vi "status.vi"(6 "tab sheet":T1(ring), 7 "TDMS File Viewer Configuration":T2) -> (3 "status":string)   [LabVIEW 2020]
uses:
  <vilib>/Utility/tdmsutil.llb/fileViewerConfigData.ctl
  <vilib>/Utility/tdmsutil.llb/TDMSFileViewerLocalizedText.vi
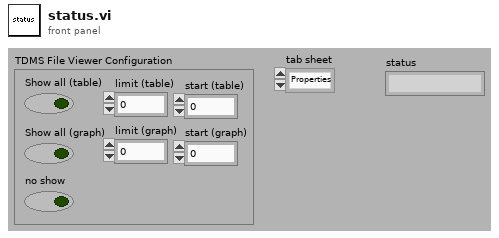
[diagram p1: front panel]
types:
  T1 = enum32{"Properties", "Values (table)", "Analog values (graph)"}
  T2 = typedef "fileViewerConfigData.ctl" = cluster{"Show all (table)":bool, "Show all (graph)":bool, "limit (table)":u64, "limit (graph)":u64, "no show":bool, "start (table)":u64, "start (graph)":u64}
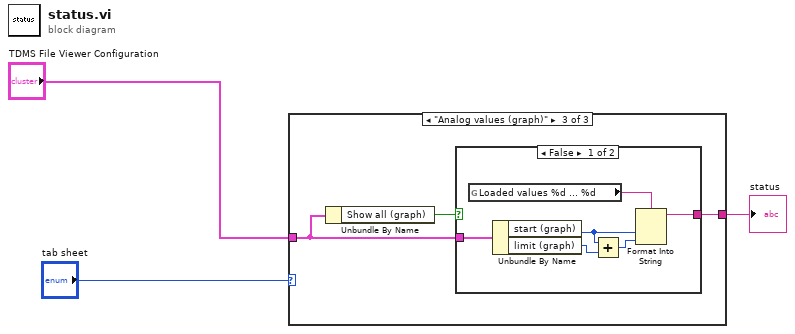
[diagram p0: block diagram]
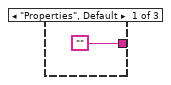
[diagram p2: hidden frame]
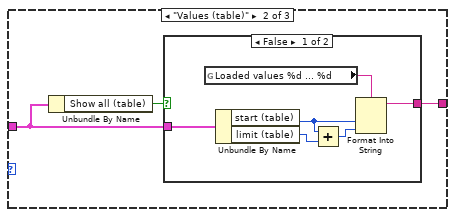
[diagram p3: hidden frame]
diagram:
  n1 = case shown="\"Analog values (graph)\"" "tab sheet" {
    tunnel: ["" w7 w16] -> w2
    tunnel: "TDMS File Viewer Configuration" -> [_ w6 w15]
    frame "Properties", Default {
    }
    frame "Values (table)" {
      n2 = Unbundle By Name(w6) -> ("Show all (table)"=w5:bool)
      n3 = case shown="False" w5 {
        tunnel: w6 -> [w13 _]
        tunnel: [w9 _] -> w7
        frame False {
          n4 = global read "TDMSFileViewerLocalizedText.vi" "Loaded values %d ... %d"() -> (w8:string)
          n5 = Unbundle By Name(w13) -> ("start (table)"=w12:u64, "limit (table)"=w11:u64)
          n6 = Add(x=w12, y=w11) -> (x+y=w10:u64)
          n7 = Format Into String(format string=w8, w12, w10) -> (resulting string=w9:string)  [unwired: 2 in, 1 out]
        }
        frame True {
        }
      }
    }
    frame "Analog values (graph)" {
      n8 = Unbundle By Name(w15) -> ("Show all (graph)"=w14:bool)
      n9 = case shown="False" w14 {
        tunnel: w15 -> [w22 _]
        tunnel: [w18 _] -> w16
        frame False {
          n10 = global read "TDMSFileViewerLocalizedText.vi" "Loaded values %d ... %d"() -> (w17:string)
          n11 = Unbundle By Name(w22) -> ("start (graph)"=w21:u64, "limit (graph)"=w20:u64)
          n12 = Add(x=w21, y=w20) -> (x+y=w19:u64)
          n13 = Format Into String(format string=w17, w21, w19) -> (resulting string=w18:string)  [unwired: 2 in, 1 out]
        }
        frame True {
        }
      }
    }
  }
  "status" <- w2
